vi "Replace Or Add Balls.vi"(10 "balls new":T1[](array[typedef]), 11 "balls":T1[](array[typedef])) -> (3 "Balls out":T1[](array[typedef]))   [LabVIEW 2017]
uses:
  <vilib>/Analysis/Matrix/Datatypes/RealMatrix.ctl
  <vilib>/Analysis/Matrix/NI_Matrix.lvlib
  SSL Detection Ball.ctl
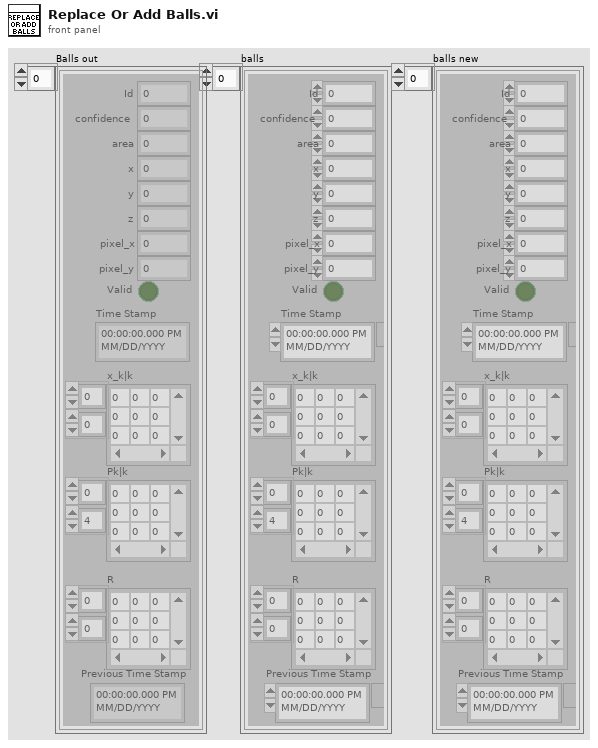
[diagram p1: front panel]
types:
  T1 = typedef "SSL Detection Ball.ctl" = cluster{"x":sgl, "area":u32, "confidence":sgl, "y":sgl, "z":sgl, "pixel_x":sgl, "pixel_y":sgl, "Valid":bool, "Time Stamp":timestamp, "x_k|k":T2, "Pk|k":T2, "Id":u32, "Previous Time Stamp":timestamp, "R":T2}
  T2 = typedef "NI_Matrix.lvlib/RealMatrix.ctl" = dbl[][]
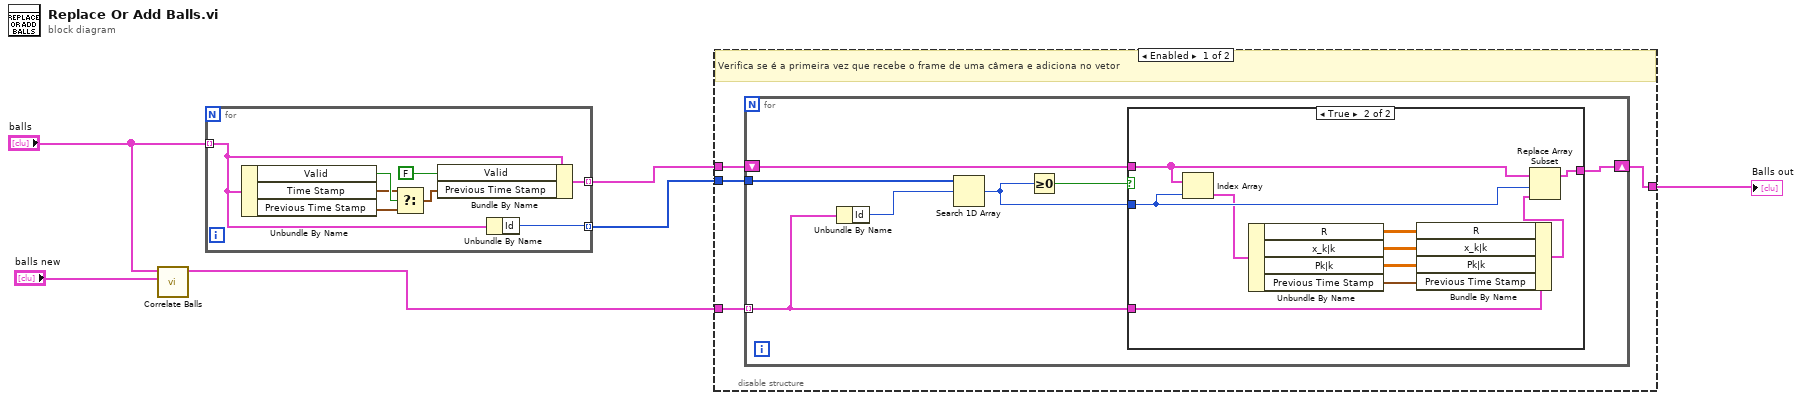
[diagram p0: block diagram]
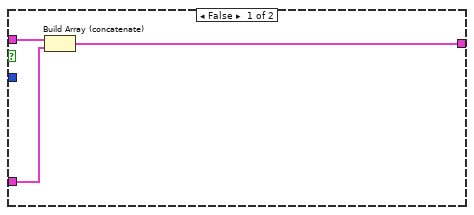
[diagram p2: hidden frame]
diagram:
  n1 = call "Correlate Balls.vi"("balls new"="balls new", "balls"="balls") -> ("balls new out"=w1:T1[])  [unwired: 9 in]
  n2 = for {
    tunnel: "balls" -> [w11] mode=indexing
    tunnel: [w14] -> w6 mode=indexing
    tunnel: [w12] -> w5 mode=indexing
    n3 = Unbundle By Name(w11) -> ("Valid"=w10:bool, "Time Stamp"=w9:timestamp, "Previous Time Stamp"=w7:timestamp)
    n4 = Select(t=w9, s=w10, f=w7) -> (s? t:f=w8:timestamp)
    n5 = Bundle By Name(cluster=w11, "Valid"=FALSE, "Previous Time Stamp"=w8) -> (w12:T1)
    n6 = Unbundle By Name(w11) -> ("Id"=w14:u32)
  }
  n7 = disable-structure "Diagram Disable Structure" shown="Enabled" {
    disable-tunnel: w5 -> [w18 _]
    disable-tunnel: w1 -> [w17 _]
    disable-tunnel: [w16 _] -> w4
    disable-tunnel: w6 -> [w15 _]
    frame Enabled {
      # "Verifica se é a primeira vez que recebe o frame de uma câmera e adiciona no vetor"
      n8 = for {
        tunnel: w17 -> [w22] mode=indexing
        tunnel: w15 -> [w23]
        shift-right: [w24] -> w16
        shift-left: w18 -> [w25]
        n9 = Unbundle By Name(w22) -> ("Id"=w21:u32)
        n10 = Search 1D Array(1D array=w23, element=w21) -> (index of element=w19:i32)  [unwired: 1 in]
        n11 = Greater Or Equal To 0?(x=w19) -> (x >= 0?=w20:bool)
        n12 = case shown="True" w20 {
          tunnel: w25 -> [w28 w37]
          tunnel: w22 -> [w26 w34]
          tunnel: [w27 w38] -> w24
          tunnel: w19 -> [_ w36]
          frame False {
            n13 = Build Array (concatenate)(w28, w26) -> (w27:T1[])
          }
          frame True {
            n14 = Index Array(array=w37, index=w36) -> (element=w35:T1)
            n15 = Unbundle By Name(w35) -> ("R"=w29:T2, "x_k|k"=w32:T2, "Pk|k"=w31:T2, "Previous Time Stamp"=w30:timestamp)
            n16 = Bundle By Name(cluster=w34, "R"=w29, "x_k|k"=w32, "Pk|k"=w31, "Previous Time Stamp"=w30) -> (w33:T1)
            n17 = Replace Array Subset(array=w37, new element=w33, index=w36) -> (w38:T1[])
          }
        }
      }
    }
    frame Disabled {
    }
  }
  "Balls out" <- w4
